vi "Array Max & Min JSON.vi"(7 "JSON Value in":refnum<class "JSON Value.lvclass">, 11 "error in (no error)":errorcluster) -> (4 "JSON Value out":refnum<class "JSON Value.lvclass">, 6 "max index":i32, 8 "JSON Value out":refnum<class "JSON Value.lvclass">, 10 "min index":i32, 15 "error out":errorcluster)   [LabVIEW 2016, in "JSON Value.lvclass"]
doc: "Finds the maximum value and minimum value of the elements in a JSON Array. The elements must all be the same literal type."
uses:
  JSON Value.lvclass
  Read Value/Read value as String.vi
  Read Value/Read value (Numeric).vi
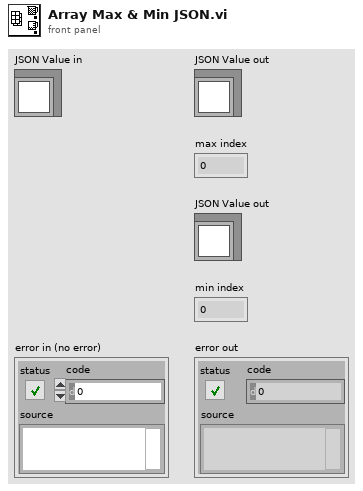
[diagram p1: front panel]
types:
  T1 = typedef "JSON Value.lvclass/JSON Types.ctl" = enum16{"String", "Numeric", "Boolean", "NULL", "Object", "Array"}
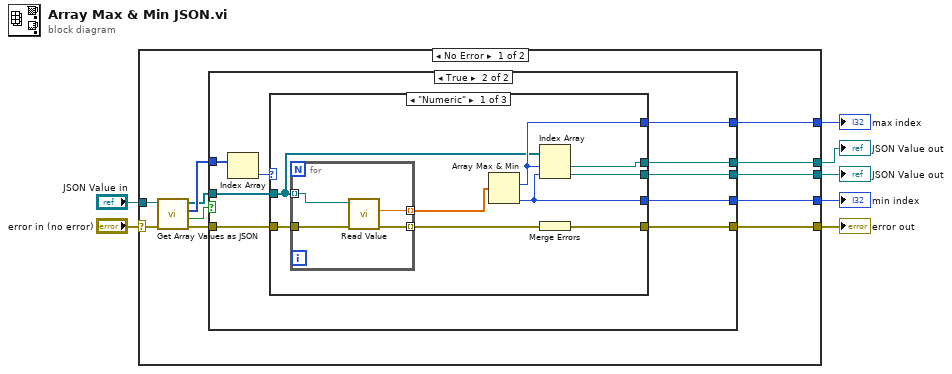
[diagram p0: block diagram]
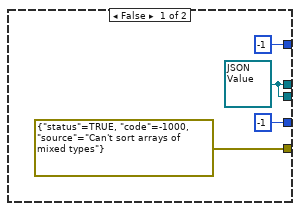
[diagram p2: hidden frame]
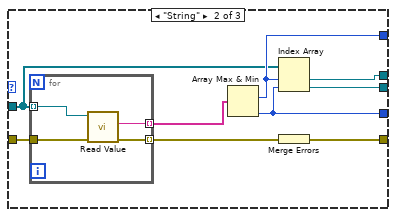
[diagram p3: hidden frame]
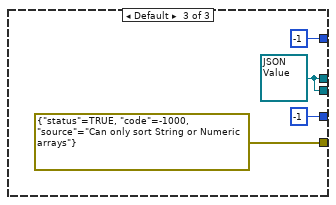
[diagram p4: hidden frame]
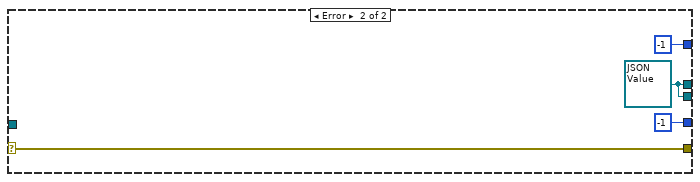
[diagram p5: hidden frame]
diagram:
  n1 = case shown="No Error" "error in (no error)" {
    selector: "error in (no error)" -> [w15 w65]
    tunnel: "JSON Value in" -> [w13 _]
    tunnel: [w18 w65] -> w5
    tunnel: [w11 w62] -> w4
    tunnel: [w10 w62] -> w3
    tunnel: [w9 -1] -> w2
    tunnel: [w8 -1] -> w1
    frame No Error {
      n2 = call "Get Array Values as JSON.vi"("error in (no error)"=w15, "JSON Value in"=w13) -> ("error out"=w14:errorcluster, "single type?"=w16:bool, "types"=w17:T1[], "values"=w12:refnum<class "JSON Value.lvclass">[])  [unwired: 6 in]
      n3 = case shown="True" w16 {
        tunnel: w12 -> [_ w31]
        tunnel: w14 -> [_ w30]
        tunnel: [errorcluster {"status"=TRUE, "code"=-1000, "source"="Can't sort arrays of mixed types"} ("error IO") w29] -> w18
        tunnel: w17 -> [_ w28]
        tunnel: [w19 w26] -> w11
        tunnel: [w19 w25] -> w10
        tunnel: [-1 w24] -> w9
        tunnel: [-1 w23] -> w8
        frame False {
          w19 = refnum<class "JSON Value.lvclass"> refnum ("JSON Object in")
        }
        frame True {
          n4 = Index Array(array=w28) -> (element=w27:T1)  [unwired: 1 in]
          n5 = case shown="\"Numeric\"" w27 {
            tunnel: w31 -> [w32 w45 _]
            tunnel: w30 -> [w40 w53 _]
            tunnel: [w37 w50 errorcluster {"status"=TRUE, "code"=-1000, "source"="Can only sort String or Numeric arrays"} ("error IO")] -> w29
            tunnel: [w36 w49 w58] -> w26
            tunnel: [w35 w48 w58] -> w25
            tunnel: [w34 w47 -1] -> w24
            tunnel: [w33 w46 -1] -> w23
            frame "Numeric" {
              n6 = for {
                tunnel: w32 -> [w41] mode=indexing
                tunnel: [w44] -> w39 mode=indexing
                tunnel: w40 -> [w43]
                tunnel: [w42] -> w38 mode=indexing
                n7 = call-poly "Read Value.vi"("error in (no error)"=w43, "JSON Numeric in"=w41) -> ("error out"=w42:errorcluster, "value"=w44:dbl)  [unwired: 8 in]
              }
              n8 = Array Max & Min(array=w39) -> (max index (indices)=w34:i32, min index (indices)=w33:i32)  [unwired: 2 out]
              n9 = Index Array(array=w32, index #1=w34, index #2=w33) -> (element #1=w36:refnum<class "JSON Value.lvclass">, element #2=w35:refnum<class "JSON Value.lvclass">)
              n10 = Merge Errors(w38) -> (w37:errorcluster)
            }
            frame "String" {
              n11 = for {
                tunnel: w45 -> [w54] mode=indexing
                tunnel: [w57] -> w52 mode=indexing
                tunnel: w53 -> [w56]
                tunnel: [w55] -> w51 mode=indexing
                n12 = call-poly "Read Value.vi"("error in (no error)"=w56, "JSON String in"=w54) -> ("error out"=w55:errorcluster, "value"=w57:string)  [unwired: 8 in]
              }
              n13 = Array Max & Min(array=w52) -> (max index (indices)=w47:i32, min index (indices)=w46:i32)  [unwired: 2 out]
              n14 = Index Array(array=w45, index #1=w47, index #2=w46) -> (element #1=w49:refnum<class "JSON Value.lvclass">, element #2=w48:refnum<class "JSON Value.lvclass">)
              n15 = Merge Errors(w51) -> (w50:errorcluster)
            }
            frame Default {
              w58 = refnum<class "JSON Value.lvclass"> refnum ("JSON Object in")
            }
          }
        }
      }
    }
    frame Error {
      w62 = refnum<class "JSON Value.lvclass"> refnum ("JSON Object in")
    }
  }
  "error out" <- w5
  "JSON Value out" <- w4
  "JSON Value out" <- w3
  "max index" <- w2
  "min index" <- w1
